vi "Connection String.vi"(8 "error in (no error)":errorcluster, 11 "MySQL in":refnum<class "MySQL.lvclass">) -> (0 "error out":errorcluster, 2 "Connected String":string, 3 "MySQL out":refnum<class "MySQL.lvclass">)   [LabVIEW 2021, in "MySQL.lvclass"]
uses:
  MySQL.lvclass
  NI_DB_API/NI_DB_API.lvclass
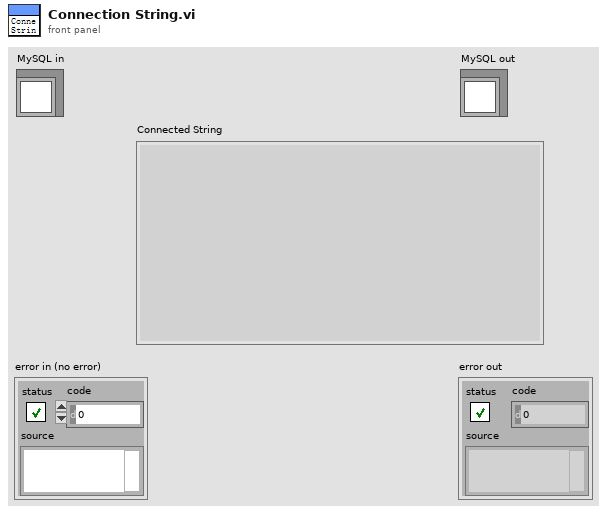
[diagram p1: front panel]
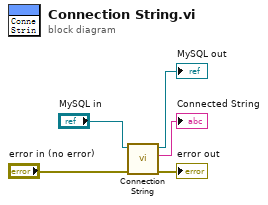
[diagram p0: block diagram]
diagram:
  n1 = call-parent "Connection String.vi"("error in (no error)"="error in (no error)", "DataBase_SQL in"="MySQL in") -> ("error out"=→"error out":errorcluster, "Connected String"=→"Connected String":string, "DataBase_SQL out"=→"MySQL out":refnum<class "MySQL.lvclass">)  [unwired: 7 in]
